vi "AO stage and shutter control.vi"() -> ()   [LabVIEW 2018]
panel:
  in  "2p shutter":refnum<k7>(container)
  in  "488 shutter":refnum<k7>(container)
  out "Numeric status":dbl
  in  "Flip Mirror":sgl(ring) items=["EMCCD Camera"=-5, "Wavefront sensor"=1]
  in  "stop":bool
  in  "baud rate (9600)":u32=9600
  in  "VISA resource name":refnum<visa-resource-name>="COM5"
  in  "Z step (10=1um)":dbl=2.0
  in  "up":bool
  in  "down":bool
  in  "XY step (10=1um)":u16=50
  in  "back":bool
  in  "front":bool
  in  "left":bool
  in  "right":bool
  # "Sample Stage"
  # "WF switch"
  # "EMCCD: -5"
  # "Wavefront Sensor: 1"
  # "Laser Shutter"
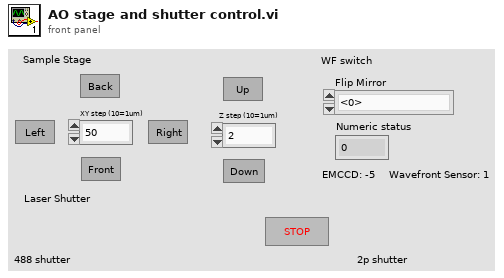
[diagram p1: front panel]
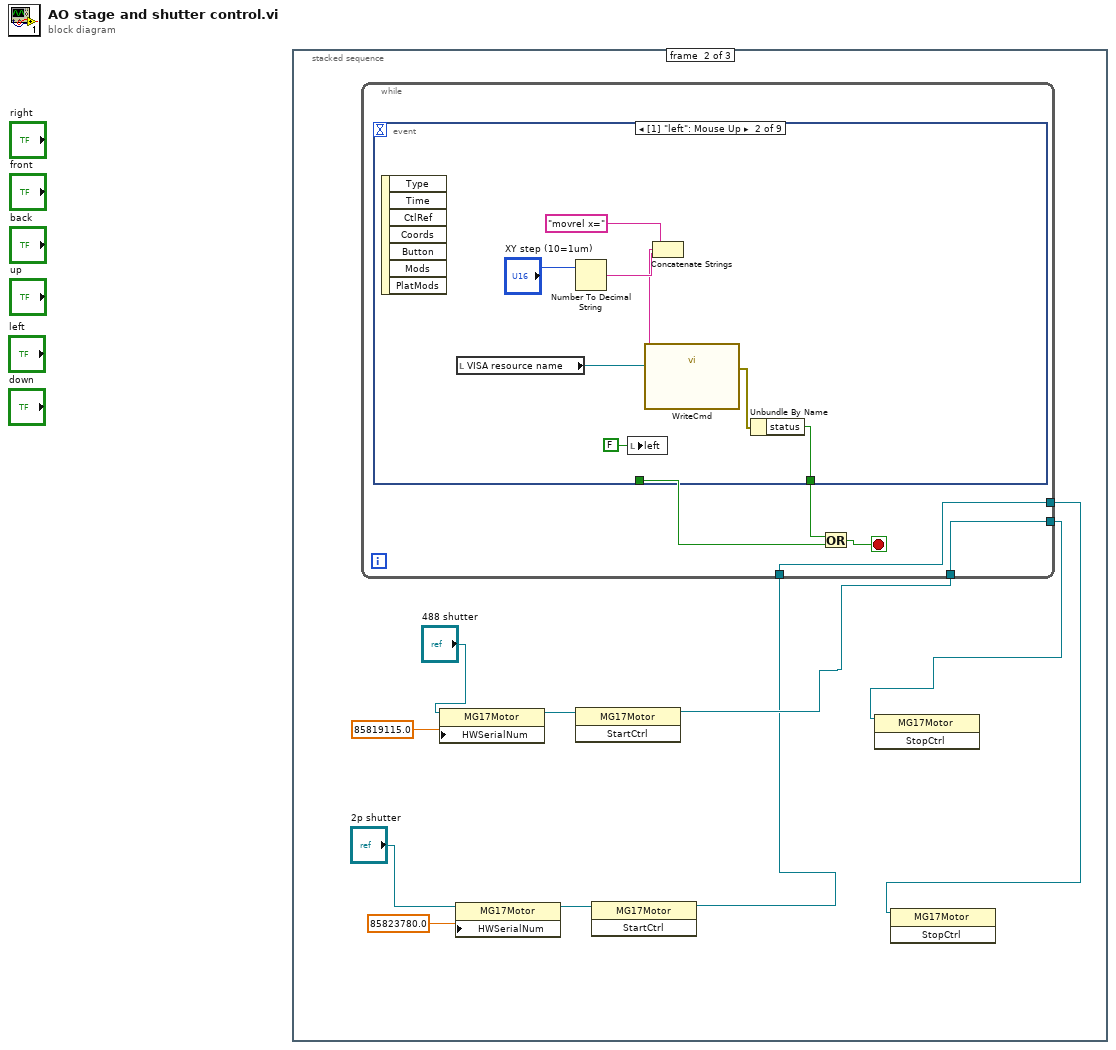
[diagram p0: block diagram]
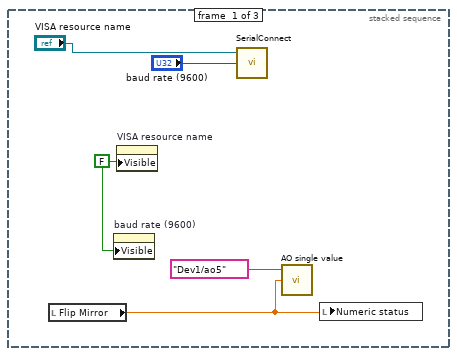
[diagram p2: hidden frame]
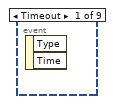
[diagram p3: hidden frame]
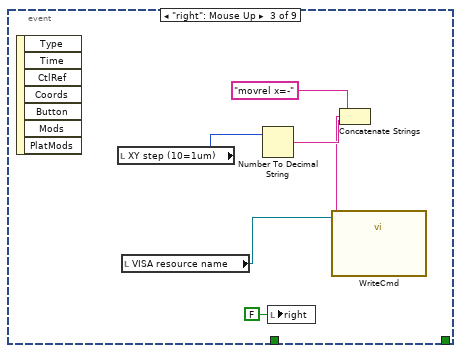
[diagram p4: hidden frame]
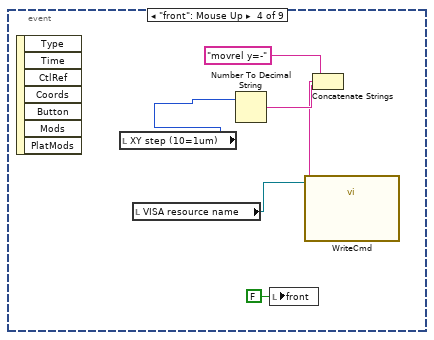
[diagram p5: hidden frame]
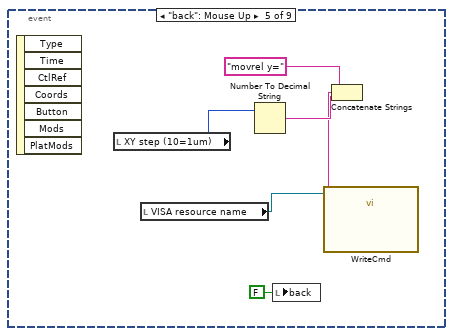
[diagram p6: hidden frame]
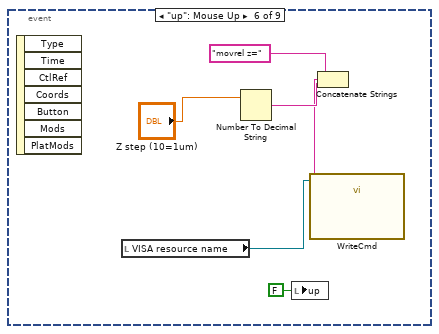
[diagram p7: hidden frame]
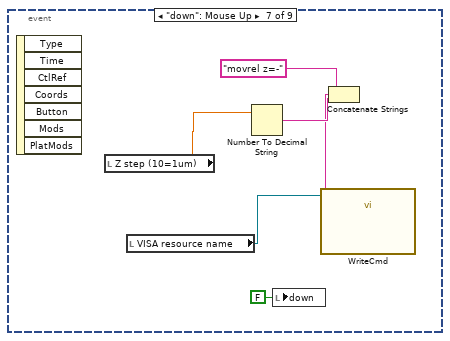
[diagram p8: hidden frame]
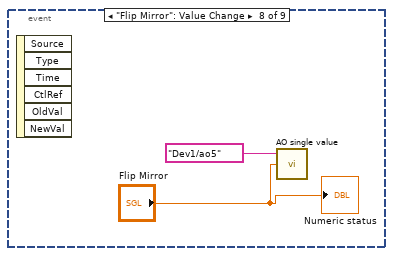
[diagram p9: hidden frame]
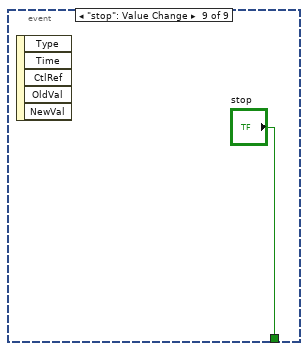
[diagram p10: hidden frame]
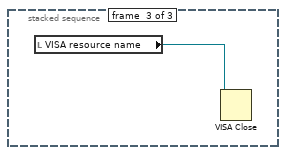
[diagram p11: hidden frame]
diagram:
  n1 = stacked-sequence {
    frame #0 {
      w3 = FALSE ("Visible")
      n2 = local read "Flip Mirror"() -> (w1:sgl)
      n3 = property on="baud rate (9600)" class="DigNum (strict)"("Visible"=w3) -> ()  [unwired: 2 in, 2 out]
      n4 = property on="VISA resource name" class="VISAName"("Visible"=w3) -> ()  [unwired: 2 in, 2 out]
      n5 = call "SerialConnect.vi"("baud rate (9600)"="baud rate (9600)", "VISA resource name"="VISA resource name") -> ()  [unwired: 1 in, 3 out]
      n6 = call "AO single value.vi"("data"=w1, "physical channels"=tag "Dev1/ao5") -> ()  [unwired: 1 in, 1 out]
      n7 = local write "Numeric status"(w1) -> ()
    }
    frame #1 {
      n8 = property class="MG17Motor"(reference="488 shutter", "HWSerialNum"=85819115.0) -> (reference out=w15:refnum<k7>)  [unwired: 1 in, 1 out]
      n9 = property class="MG17Motor"(reference="2p shutter", "HWSerialNum"=85823780.0) -> (reference out=w10:refnum<k7>)  [unwired: 1 in, 1 out]
      n10 = invoke class="MG17Motor" method="StartCtrl"(reference=w15) -> (reference out=w14:refnum<k7>)  [unwired: 2 in, 2 out]
      n11 = invoke class="MG17Motor" method="StartCtrl"(reference=w10) -> (reference out=w7:refnum<k7>)  [unwired: 2 in, 2 out]
      n12 = while {
        tunnel: w14 -> [w17]
        tunnel: [w17] -> w13
        tunnel: w7 -> [w16]
        tunnel: [w16] -> w6
        stop <- w20 stop-if-true
        n13 = event shown="[1] \"left\": Mouse Up" {
          selector: _ -> [_ _ _ _ _ _ _ _ _]
          dyn-events: _ -> [_ _ _ _ _ _ _ _ _]
          timeout: _ -> [_ _ _ _ _ _ _ _ _]
          tunnel: [_ _ _ _ _ _ _ _ "stop"] -> w19
          tunnel: [_ w21 _ _ _ _ _ _ _] -> w18
          event Timeout {
            n14 = event-data() -> ()  [unwired: 1 in, 2 out]
          }
          event "left": Mouse Up {
            n15 = event-data() -> ()  [unwired: 1 in, 7 out]
            n16 = local read "VISA resource name"() -> (w24:refnum<visa-resource-name>)
            n17 = Number To Decimal String(number="XY step (10=1um)") -> (decimal integer string=w26:string)  [unwired: 1 in]
            n18 = local write "left"(FALSE ("left")) -> ()
            n19 = Concatenate Strings("movrel x=", w26) -> (w25:string)
            n20 = call "WriteCmd.vi"("Command"=w25, "VISA resource name"=w24) -> ("error"=w22:errorcluster)  [unwired: 1 in]
            n21 = Unbundle By Name(w22) -> ("status"=w21:bool)
          }
          event "right": Mouse Up {
            n22 = event-data() -> ()  [unwired: 1 in, 7 out]
            n23 = local read "XY step (10=1um)"() -> (w29:u16)
            n24 = local read "VISA resource name"() -> (w31:refnum<visa-resource-name>)
            n25 = Number To Decimal String(number=w29) -> (decimal integer string=w33:string)  [unwired: 1 in]
            n26 = local write "right"(FALSE ("right")) -> ()
            n27 = Concatenate Strings("movrel x=-", w33) -> (w32:string)
            n28 = call "WriteCmd.vi"("Command"=w32, "VISA resource name"=w31) -> ()  [unwired: 1 in, 1 out]
          }
          event "front": Mouse Up {
            n29 = event-data() -> ()  [unwired: 1 in, 7 out]
            n30 = local read "XY step (10=1um)"() -> (w35:u16)
            n31 = local read "VISA resource name"() -> (w37:refnum<visa-resource-name>)
            n32 = Number To Decimal String(number=w35) -> (decimal integer string=w39:string)  [unwired: 1 in]
            n33 = local write "front"(FALSE ("front")) -> ()
            n34 = Concatenate Strings("movrel y=-", w39) -> (w38:string)
            n35 = call "WriteCmd.vi"("Command"=w38, "VISA resource name"=w37) -> ()  [unwired: 1 in, 1 out]
          }
          event "back": Mouse Up {
            n36 = event-data() -> ()  [unwired: 1 in, 7 out]
            n37 = local read "XY step (10=1um)"() -> (w41:u16)
            n38 = local read "VISA resource name"() -> (w43:refnum<visa-resource-name>)
            n39 = Number To Decimal String(number=w41) -> (decimal integer string=w45:string)  [unwired: 1 in]
            n40 = local write "back"(FALSE ("back")) -> ()
            n41 = Concatenate Strings("movrel y=", w45) -> (w44:string)
            n42 = call "WriteCmd.vi"("Command"=w44, "VISA resource name"=w43) -> ()  [unwired: 1 in, 1 out]
          }
          event "up": Mouse Up {
            n43 = event-data() -> ()  [unwired: 1 in, 7 out]
            n44 = local read "VISA resource name"() -> (w49:refnum<visa-resource-name>)
            n45 = Number To Decimal String(number="Z step (10=1um)") -> (decimal integer string=w51:string)  [unwired: 1 in]
            n46 = local write "up"(FALSE ("up")) -> ()
            n47 = Concatenate Strings("movrel z=", w51) -> (w50:string)
            n48 = call "WriteCmd.vi"("Command"=w50, "VISA resource name"=w49) -> ()  [unwired: 1 in, 1 out]
          }
          event "down": Mouse Up {
            n49 = event-data() -> ()  [unwired: 1 in, 7 out]
            n50 = local read "Z step (10=1um)"() -> (w53:dbl)
            n51 = local read "VISA resource name"() -> (w55:refnum<visa-resource-name>)
            n52 = Number To Decimal String(number=w53) -> (decimal integer string=w57:string)  [unwired: 1 in]
            n53 = local write "down"(FALSE ("down")) -> ()
            n54 = Concatenate Strings("movrel z=-", w57) -> (w56:string)
            n55 = call "WriteCmd.vi"("Command"=w56, "VISA resource name"=w55) -> ()  [unwired: 1 in, 1 out]
          }
          event "Flip Mirror": Value Change {
            n56 = event-data() -> ()  [unwired: 1 in, 6 out]
            n57 = call "AO single value.vi"("data"="Flip Mirror", "physical channels"=tag "Dev1/ao5") -> ()  [unwired: 1 in, 1 out]
            "Numeric status" <- "Flip Mirror"
          }
          event "stop": Value Change {
            n58 = event-data() -> ()  [unwired: 1 in, 5 out]
          }
        }
        n59 = Or(x=w18, y=w19) -> (x .or. y?=w20:bool)
      }
      n60 = invoke class="MG17Motor" method="StopCtrl"(reference=w13) -> ()  [unwired: 2 in, 3 out]
      n61 = invoke class="MG17Motor" method="StopCtrl"(reference=w6) -> ()  [unwired: 2 in, 3 out]
    }
    frame #2 {
      n62 = local read "VISA resource name"() -> (w62:refnum<visa-resource-name>)
      n63 = VISA Close(VISA resource name=w62) -> ()  [unwired: 1 in, 1 out]
    }
  }
